vi "New Chart.vi"(8 "Error In":errorcluster) -> (0 "Error Out":errorcluster, 3 "New LQChart":refnum<class "LQChart.lvclass">)   [LabVIEW 2013]
uses:
  src/LabVIEW/LQ Extras/LQChart/LQChart.lvclass
  Global Chart List Action.ctl
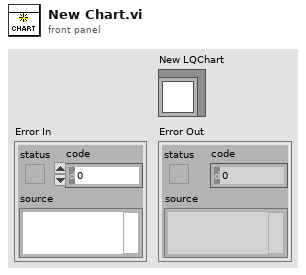
[diagram p1: front panel]
types:
  T1 = typedef "Global Chart List Action.ctl" = enum16{"Clear", "Register Chart", "Append to Charts"}
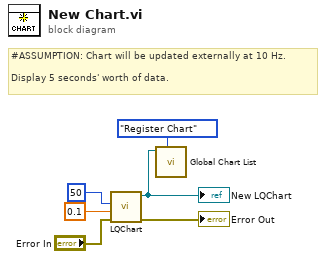
[diagram p0: block diagram]
diagram:
  # "#ASSUMPTION: Chart will be updated externally at 10 Hz.\n\nDisplay 5 seconds' worth of data."
  n1 = call "LQChart.vi"("Error In"="Error In", "xMultiplier"=0.1, "historyLength"=50) -> ("Error Out"=→"Error Out":errorcluster, "New LQChart"=w4:refnum<class "LQChart.lvclass">)  [unwired: 7 in]
  "New LQChart" <- w4
  n2 = call "Global Chart List.vi"("Action"=Global_Chart_List_Action."Register Chart", "Chart Ref"=w4) -> ()  [unwired: 10 in]
